vi "save AlarmList database.vi"(8 "error in (no error)":errorcluster, 11 "project":T3) -> (0 "error out":errorcluster)   [LabVIEW 2016, in "opSignIn.lvlib"]
uses:
  opSignIn.lvlib
  AlarmList.ctl
  solutionList.ctl
  <vilib>/Utility/VariantDataType/VariantType.lvlib
panel:
  in  "solutionList":T1
  in  "alarmList":T2
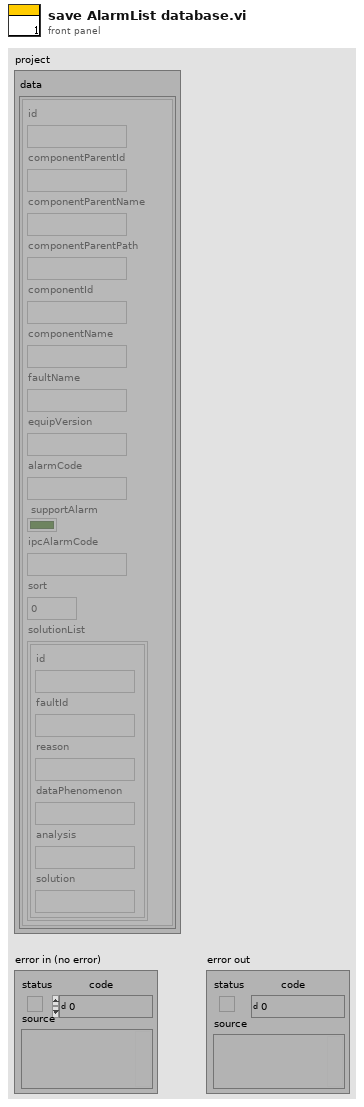
[diagram p1: front panel]
types:
  T1 = typedef "opSignIn.lvlib/solutionList.ctl" = cluster{"id":string, "faultId":string, "reason":string, "dataPhenomenon":string, "analysis":string, "solution":string, "alarmListId":string}
  T2 = typedef "opSignIn.lvlib/AlarmList.ctl" = cluster{"id":string, "componentParentId":string, "componentParentName":string, "componentParentPath":string, "componentId":string, "componentName":string, "faultName":string, "equipVersion":string, "alarmCode":string, "supportAlarm":bool, "ipcAlarmCode":string, "sort":i32}
  T3 = typedef "opSignIn.lvlib/报警格式.ctl" = cluster{"data":T4[]}
  T4 = typedef "opSignIn.lvlib/元素.ctl" = cluster{"id":string, "componentParentId":string, "componentParentName":string, "componentParentPath":string, "componentId":string, "componentName":string, "faultName":string, "equipVersion":string, "alarmCode":string, "supportAlarm":bool, "ipcAlarmCode":string, "sort":dbl, "solutionList":cluster{"id":string, "faultId":string, "reason":string, "dataPhenomenon":string, "analysis":string, "solution":string}[]}
  T5 = cluster{"id":string, "faultId":string, "reason":string, "dataPhenomenon":string, "analysis":string, "solution":string}[]
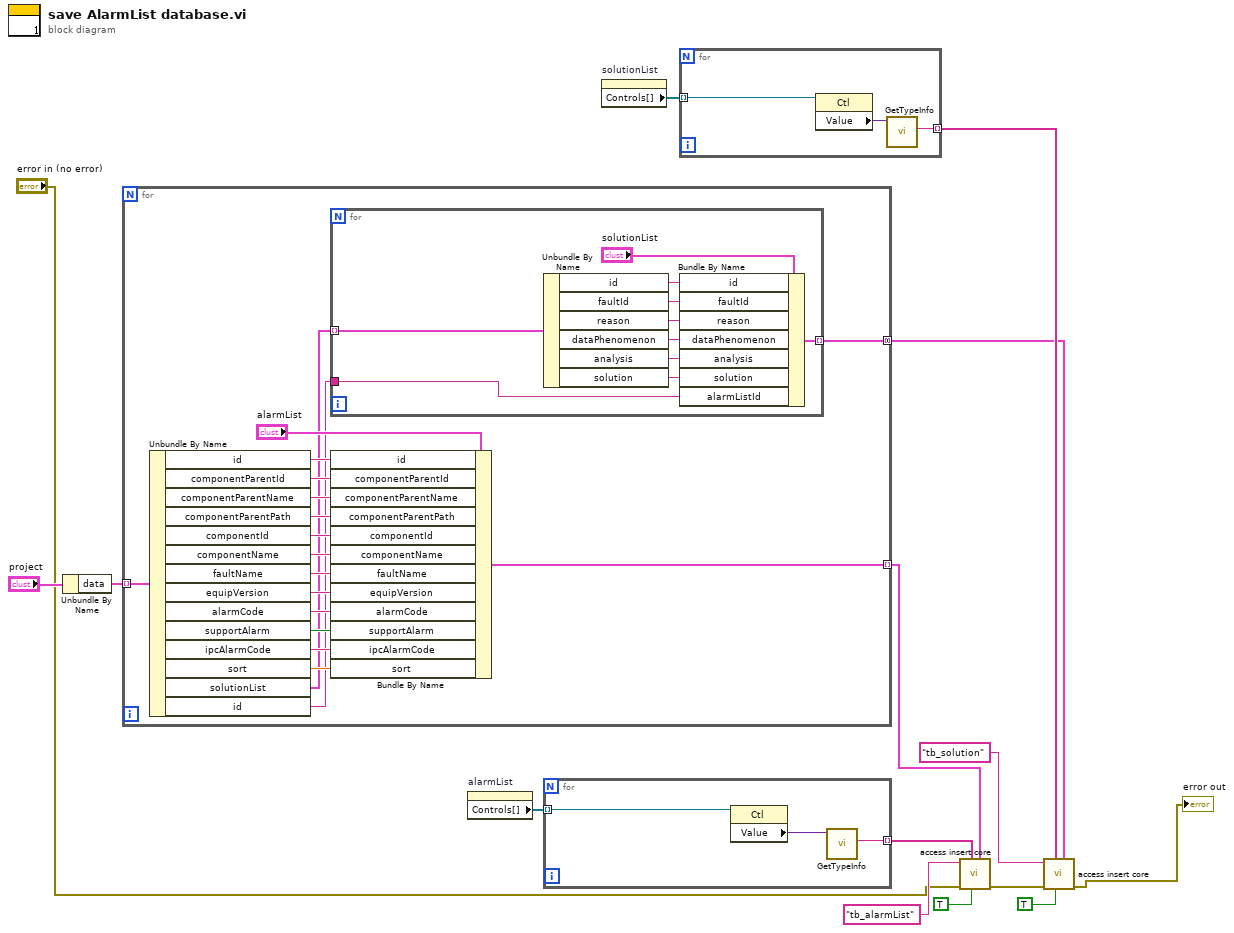
[diagram p0: block diagram]
diagram:
  n1 = Unbundle By Name("project") -> ("data"=w14:T4[])
  n2 = for {
    tunnel: w14 -> [w33] mode=indexing
    tunnel: [w17] -> w13 mode=indexing
    tunnel: [w16] -> w4 mode=concatenating
    n3 = Unbundle By Name(w33) -> ("id"=w31:string, "componentParentId"=w30:string, "componentParentName"=w29:string, "componentParentPath"=w28:string, "componentId"=w27:string, "componentName"=w26:string, "faultName"=w25:string, "equipVersion"=w24:string, "alarmCode"=w23:string, "supportAlarm"=w22:bool, "ipcAlarmCode"=w21:string, "sort"=w20:dbl, "solutionList"=w18:T5, "id"=w19:string)
    n4 = for {
      tunnel: w18 -> [w43] mode=indexing
      tunnel: w19 -> [w35]
      tunnel: [w34] -> w16 mode=indexing
      n5 = Unbundle By Name(w43) -> ("id"=w41:string, "faultId"=w40:string, "reason"=w39:string, "dataPhenomenon"=w38:string, "analysis"=w37:string, "solution"=w36:string)
      n6 = Bundle By Name(cluster="solutionList", "id"=w41, "faultId"=w40, "reason"=w39, "dataPhenomenon"=w38, "analysis"=w37, "solution"=w36, "alarmListId"=w35) -> (w34:T1)
    }
    n7 = Bundle By Name(cluster="alarmList", "id"=w31, "componentParentId"=w30, "componentParentName"=w29, "componentParentPath"=w28, "componentId"=w27, "componentName"=w26, "faultName"=w25, "equipVersion"=w24, "alarmCode"=w23, "supportAlarm"=w22, "ipcAlarmCode"=w21, "sort"=w20) -> (w17:T2)
  }
  n8 = property on="alarmList" class="Clust (严格)"() -> ("Controls[]"=w12:refnum<vi>[])  [unwired: 2 in, 2 out]
  n9 = for {
    tunnel: w12 -> [w45] mode=indexing
    tunnel: [w46] -> w11 mode=indexing
    n10 = property class="Ctl"(reference=w45) -> ("Value"=w44:variant)  [unwired: 1 in, 2 out]
    n11 = call <vilib>:"GetTypeInfo.vi"("Variant"=w44) -> ("Name"=w46:string)  [unwired: 6 in, 4 out]
  }
  n12 = property on="solutionList" class="Clust (严格)"() -> ("Controls[]"=w6:refnum<vi>[])  [unwired: 2 in, 2 out]
  n13 = for {
    tunnel: w6 -> [w48] mode=indexing
    tunnel: [w49] -> w5 mode=indexing
    n14 = property class="Ctl"(reference=w48) -> ("Value"=w47:variant)  [unwired: 1 in, 2 out]
    n15 = call <vilib>:"GetTypeInfo.vi"("Variant"=w47) -> ("Name"=w49:string)  [unwired: 6 in, 4 out]
  }
  n16 = call "access insert core.vi"("data"=w13, "delete table?"=TRUE, "columns"=w11, "error in (no error)"="error in (no error)", "table"="tb_alarmList") -> ("error out"=w8:errorcluster)  [unwired: 6 in]
  n17 = call "access insert core.vi"("data"=w4, "delete table?"=TRUE, "columns"=w5, "error in (no error)"=w8, "table"="tb_solution") -> ("error out"=→"error out":errorcluster)  [unwired: 6 in]
